vi "MARATHON_CHARGING1.vi"() -> ()   [LabVIEW 2018]
uses:
  <userlib>/LV-Link3/PolySubVIs/DtOLTimingSetInput.vi
  <userlib>/LV-Link3/PolySubVIs/DtOLReadMultiple2D.vi
panel:
  out "Waveform Graph":dbl[](graph)
  out "Transition Time":dbl format="%<%H:%M:%S>t"
  out "Array":bool[](array[boolean])
  in  "Limit Batt Voltage":dbl[](array[numeric]) format="%_4g"
  in  "Limit Cell Voltage":dbl[](array[numeric]) format="%_3g"
  out "x+y 2":dbl[](array[numeric])
  out "x+y":dbl[](array[knob]) scale=0.0..32.0
  out "Time 20":dbl format="%<%H:%M:%S>t"
  out "Time 19":dbl format="%<%H:%M:%S>t"
  out "Time 18":dbl format="%<%H:%M:%S>t"
  out "Time 17":dbl format="%<%H:%M:%S>t"
  out "Time 16":dbl format="%<%H:%M:%S>t"
  out "Time 15":dbl format="%<%H:%M:%S>t"
  out "Time 14":dbl format="%<%H:%M:%S>t"
  out "Time 13":dbl format="%<%H:%M:%S>t"
  out "Time 12":dbl format="%<%H:%M:%S>t"
  out "Time 11":dbl format="%<%H:%M:%S>t"
  out "Time 10":dbl format="%<%H:%M:%S>t"
  out "Time 9":dbl format="%<%H:%M:%S>t"
  out "Time 8":dbl format="%<%H:%M:%S>t"
  out "Time 7":dbl format="%<%H:%M:%S>t"
  out "Time 6":dbl format="%<%H:%M:%S>t"
  out "Time 5":dbl format="%<%H:%M:%S>t"
  out "Time 4":dbl format="%<%H:%M:%S>t"
  out "Time 3":dbl format="%<%H:%M:%S>t"
  out "Time 2":dbl format="%<%H:%M:%S>t"
  out "Time 1":dbl format="%<%H:%M:%S>t"
  out "CELL #19":bool[](array[boolean])
  out "CELL #20":bool[](array[boolean])
  out "CELL #18":bool[](array[boolean])
  out "CELL #17":bool[](array[boolean])
  out "CELL #16":bool[](array[boolean])
  out "CELL #15":bool[](array[boolean])
  out "CELL #14":bool[](array[boolean])
  out "CELL #13":bool[](array[boolean])
  out "CELL #12":bool[](array[boolean])
  out "CELL #11":bool[](array[boolean])
  out "CELL #10":bool[](array[boolean])
  out "CELL #9":bool[](array[boolean])
  out "CELL #8":bool[](array[boolean])
  out "CELL #7":bool[](array[boolean])
  out "CELL #6":bool[](array[boolean])
  out "CELL #5":bool[](array[boolean])
  out "CELL #4":bool[](array[boolean])
  out "CELL #3":bool[](array[boolean])
  out "CELL #2":bool[](array[boolean])
  out "CELL #1":bool[](array[boolean])
  out "VOLT # 20":dbl[](array[numeric])
  out "VOLT # 19":dbl[](array[numeric])
  out "VOLT # 18":dbl[](array[numeric])
  out "VOLT # 17":dbl[](array[numeric])
  out "VOLT # 16":dbl[](array[numeric])
  out "VOLT # 15":dbl[](array[numeric])
  out "VOLT # 14":dbl[](array[numeric])
  out "VOLT # 13":dbl[](array[numeric])
  out "VOLT # 12":dbl[](array[numeric])
  out "VOLT # 11":dbl[](array[numeric])
  out "VOLT # 10":dbl[](array[numeric])
  out "VOLT # 9":dbl[](array[numeric])
  out "VOLT # 8":dbl[](array[numeric])
  out "VOLT # 7":dbl[](array[numeric])
  out "VOLT # 6":dbl[](array[numeric])
  out "VOLT # 5":dbl[](array[numeric])
  out "VOLT # 4":dbl[](array[numeric])
  out "VOLT # 3":dbl[](array[numeric])
  out "VOLT # 2":dbl[](array[numeric])
  out "VOLT # 1":dbl[](array[numeric])
  in  "POWER":bool caption="START"
  in  "stop":bool
  # "FLUKE"
  # "179 Multimeter"
  # "28.56789 VOLTS"
  # "Hold"
  # "Range"
  # "ON"
  # "SuperMasterCharger"
  # "R"
  # "mV"
  # "Current"
  # "Time"
  # "000.7"
  # "04:56"
  # "D"
  # "V--"
  # "20 CELLS"
  # "Voltage"
  # "A--"
  # "OFF"
  # "STATUS"
  # "CHARGING"
  # "WATER"
  # "Jfm"
  # "ACID"
  # "1"
  # "Run"
  # "2"
  # "3"
  # "M"
  # "T"
  # "4"
  # "6"
  # "B"
  # "ST"
  # "5"
  # "CU"
  # "SAFT"
  # "8"
  # "OPT"
  # "V"
  # "RST"
  # "7"
  # "9"
  # "Vie"
  # "FN"
  # "ENT"
  # "0"
  # "C"
  # "P"
  # "POWER"
  # "Harness"
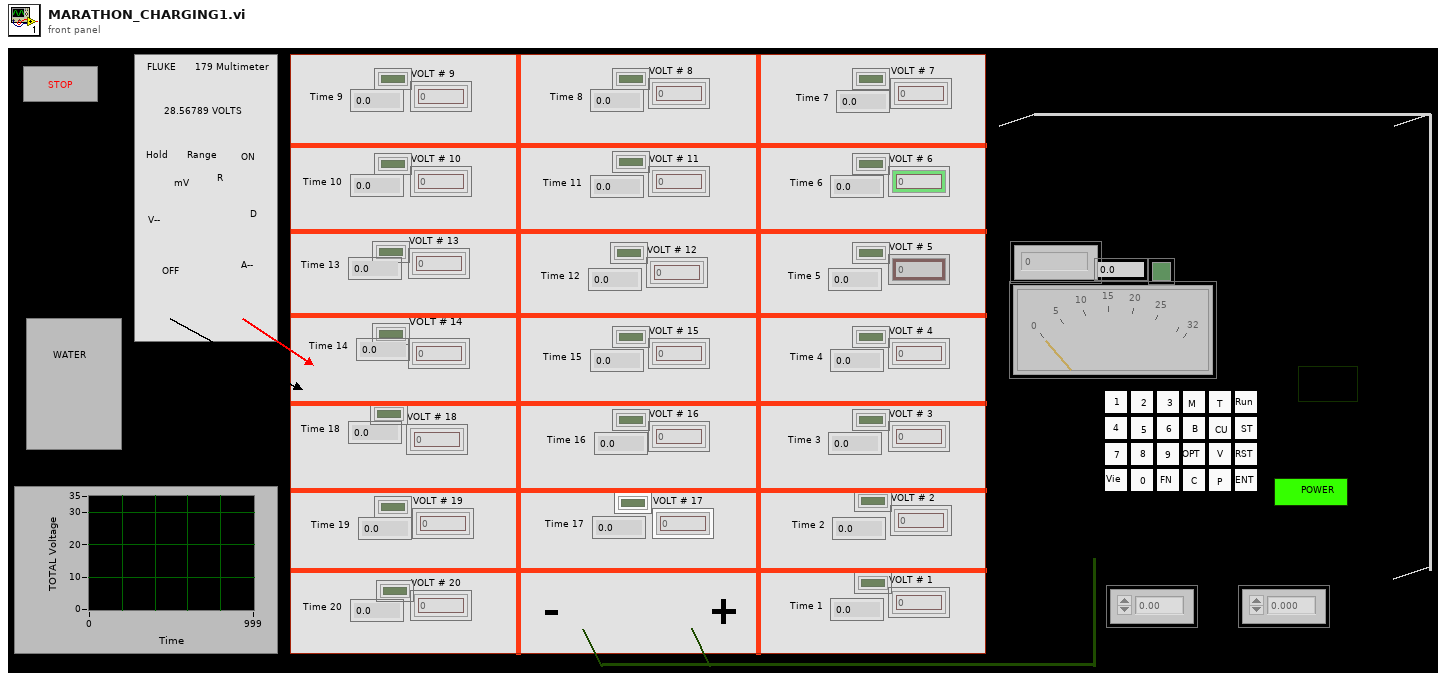
[diagram p1: front panel]
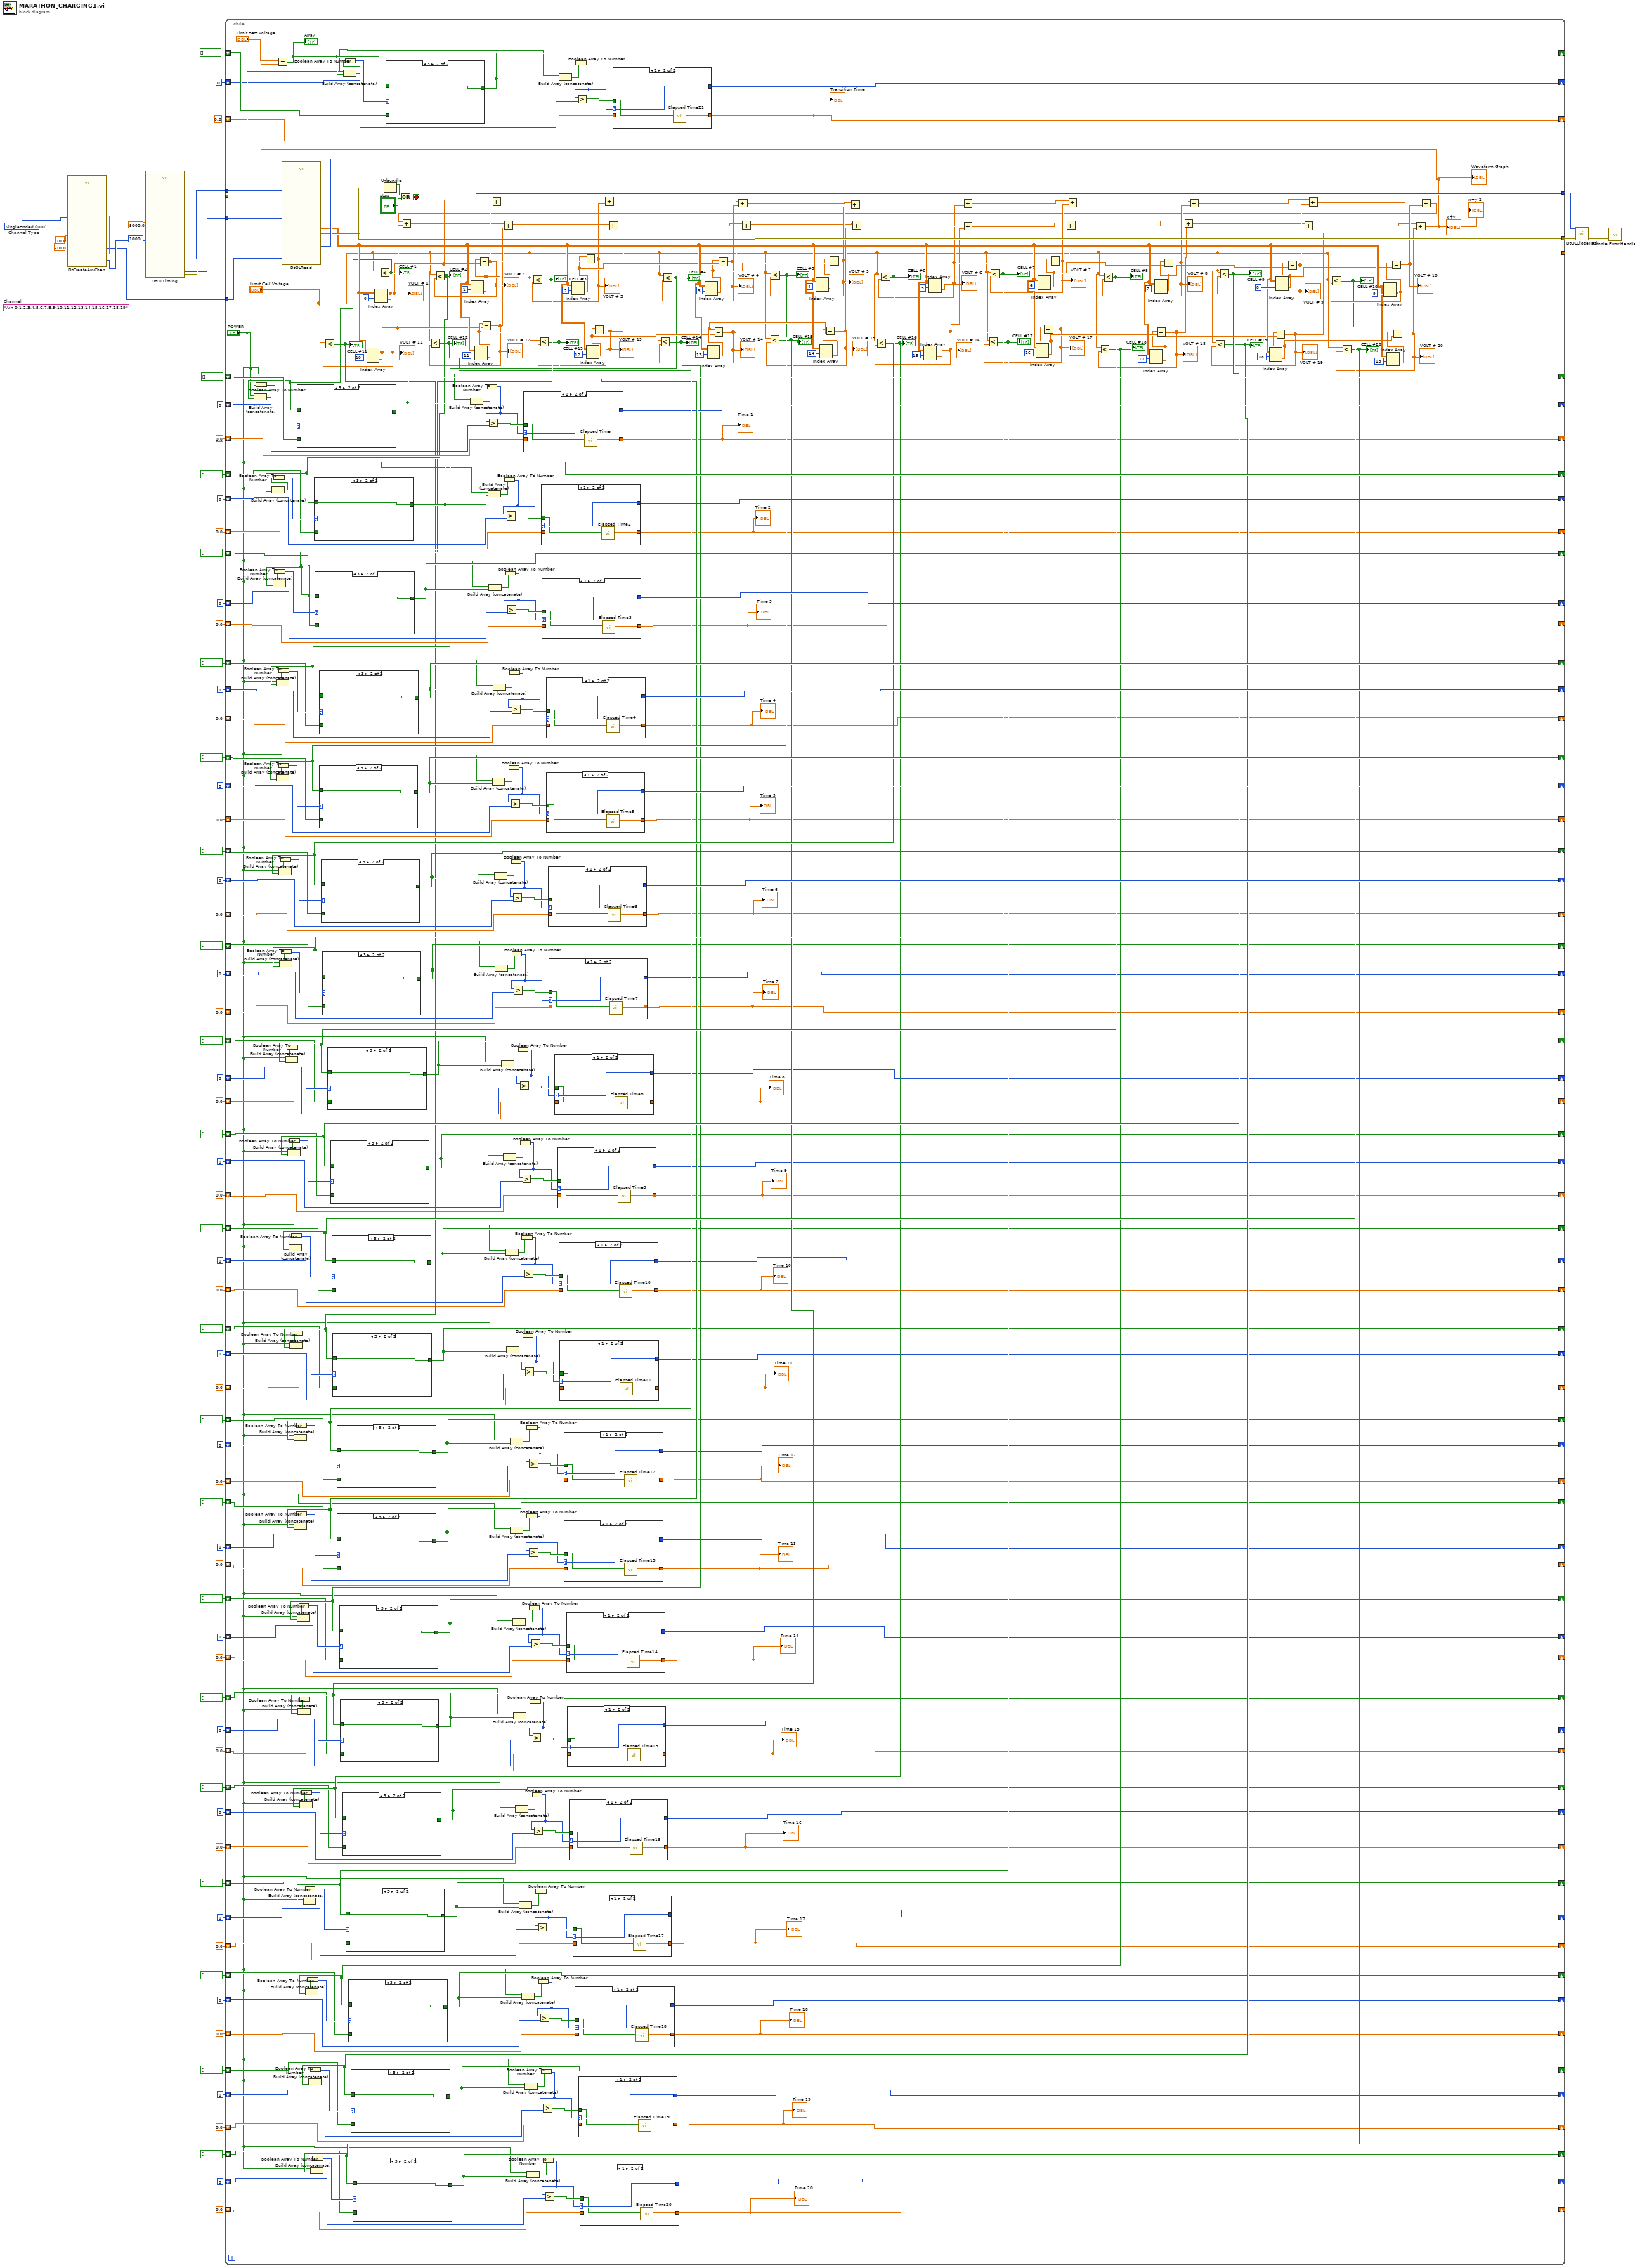
[diagram p0: block diagram]
diagram:
  w78 = 100 items=["Differential"=101, "SingleEnded"=100]  # Channel Type
  w75 = "Ain 0,1,2,3,4,5,6,7,8,9,10,11,12,13,14,15,16,17,18,19"  # Channel
  n1 = call <userlib>:"DtCreateAinChan.vi"("Channel Type"=w78, "Range Min"=-10.0, "Range Max"=10.0, "Channel"=w75) -> ("Task out"=w65:i32, "Actual Number of Channels"=w64:u32, "error out"=w74:errorcluster)  [unwired: 9 in]
  n2 = call-poly <userlib>:"DtOLTiming.vi"("Samples Per Channel"=u32 1000, "error in (no error)"=w74, "Sample Freq (Hz)"=5000.0, "Task in"=w65) -> ("error out"=w71:errorcluster, "Buffer Size"=w70:u32, "Task out"=w69:i32)  [unwired: 4 in, 1 out]
  n3 = while {
    tunnel: w71 -> [w418]
    tunnel: w70 -> [w416]
    tunnel: w69 -> [w417]
    tunnel: [w413] -> w68
    tunnel: [w414] -> w67
    tunnel: w64 -> [w412]
    shift-right: [w271] -> _
    shift-left: bool[] [] -> [w370]
    shift-right: [w230] -> _
    shift-left: u32 0 -> [w369]
    shift-right: [w117] -> _
    shift-left: 0.0 ("Elapsed Time (s)") -> [w368]
    shift-right: [w270] -> _
    shift-left: bool[] [] -> [w269]
    shift-right: [w267] -> _
    shift-left: u32 0 -> [w266]
    shift-right: [w99] -> _
    shift-left: 0.0 ("Elapsed Time (s)") -> [w265]
    shift-right: [w264] -> _
    shift-left: bool[] [] -> [w263]
    shift-right: [w262] -> _
    shift-left: u32 0 -> [w261]
    shift-right: [w98] -> _
    shift-left: 0.0 ("Elapsed Time (s)") -> [w260]
    shift-right: [w259] -> _
    shift-left: bool[] [] -> [w258]
    shift-right: [w257] -> _
    shift-left: u32 0 -> [w256]
    shift-right: [w96] -> _
    shift-left: 0.0 ("Elapsed Time (s)") -> [w255]
    shift-right: [w254] -> _
    shift-left: bool[] [] -> [w252]
    shift-right: [w253] -> _
    shift-left: u32 0 -> [w251]
    shift-right: [w95] -> _
    shift-left: 0.0 ("Elapsed Time (s)") -> [w250]
    shift-right: [w249] -> _
    shift-left: bool[] [] -> [w248]
    shift-right: [w247] -> _
    shift-left: u32 0 -> [w246]
    shift-right: [w94] -> _
    shift-left: 0.0 ("Elapsed Time (s)") -> [w245]
    shift-right: [w222] -> _
    shift-left: bool[] [] -> [w221]
    shift-right: [w220] -> _
    shift-left: u32 0 -> [w219]
    shift-right: [w93] -> _
    shift-left: 0.0 ("Elapsed Time (s)") -> [w218]
    shift-right: [w217] -> _
    shift-left: bool[] [] -> [w191]
    shift-right: [w216] -> _
    shift-left: u32 0 -> [w190]
    shift-right: [w92] -> _
    shift-left: 0.0 ("Elapsed Time (s)") -> [w189]
    shift-right: [w215] -> _
    shift-left: bool[] [] -> [w188]
    shift-right: [w214] -> _
    shift-left: u32 0 -> [w187]
    shift-right: [w91] -> _
    shift-left: 0.0 ("Elapsed Time (s)") -> [w186]
    shift-right: [w213] -> _
    shift-left: bool[] [] -> [w185]
    shift-right: [w212] -> _
    shift-left: u32 0 -> [w184]
    shift-right: [w90] -> _
    shift-left: 0.0 ("Elapsed Time (s)") -> [w183]
    shift-right: [w211] -> _
    shift-left: bool[] [] -> [w182]
    shift-right: [w210] -> _
    shift-left: u32 0 -> [w181]
    shift-right: [w89] -> _
    shift-left: 0.0 ("Elapsed Time (s)") -> [w180]
    shift-right: [w209] -> _
    shift-left: bool[] [] -> [w179]
    shift-right: [w208] -> _
    shift-left: u32 0 -> [w178]
    shift-right: [w88] -> _
    shift-left: 0.0 ("Elapsed Time (s)") -> [w177]
    shift-right: [w207] -> _
    shift-left: bool[] [] -> [w176]
    shift-right: [w206] -> _
    shift-left: u32 0 -> [w175]
    shift-right: [w87] -> _
    shift-left: 0.0 ("Elapsed Time (s)") -> [w174]
    shift-right: [w205] -> _
    shift-left: bool[] [] -> [w173]
    shift-right: [w204] -> _
    shift-left: u32 0 -> [w172]
    shift-right: [w86] -> _
    shift-left: 0.0 ("Elapsed Time (s)") -> [w171]
    shift-right: [w203] -> _
    shift-left: bool[] [] -> [w170]
    shift-right: [w202] -> _
    shift-left: u32 0 -> [w169]
    shift-right: [w85] -> _
    shift-left: 0.0 ("Elapsed Time (s)") -> [w168]
    shift-right: [w201] -> _
    shift-left: bool[] [] -> [w167]
    shift-right: [w200] -> _
    shift-left: u32 0 -> [w166]
    shift-right: [w84] -> _
    shift-left: 0.0 ("Elapsed Time (s)") -> [w165]
    shift-right: [w199] -> _
    shift-left: bool[] [] -> [w164]
    shift-right: [w198] -> _
    shift-left: u32 0 -> [w163]
    shift-right: [w83] -> _
    shift-left: 0.0 ("Elapsed Time (s)") -> [w162]
    shift-right: [w197] -> _
    shift-left: bool[] [] -> [w161]
    shift-right: [w196] -> _
    shift-left: u32 0 -> [w160]
    shift-right: [w82] -> _
    shift-left: 0.0 ("Elapsed Time (s)") -> [w159]
    shift-right: [w195] -> _
    shift-left: bool[] [] -> [w158]
    shift-right: [w194] -> _
    shift-left: u32 0 -> [w157]
    shift-right: [w81] -> _
    shift-left: 0.0 ("Elapsed Time (s)") -> [w156]
    shift-right: [w193] -> _
    shift-left: bool[] [] -> [w155]
    shift-right: [w192] -> _
    shift-left: u32 0 -> [w154]
    shift-right: [w80] -> _
    shift-left: 0.0 ("Elapsed Time (s)") -> [w153]
    tunnel: ["Limit Cell Voltage"] -> _
    shift-right: [w105] -> _
    shift-left: bool[] [] -> [w104]
    shift-right: [w102] -> _
    shift-left: u32 0 -> [w101]
    shift-right: [w97] -> _
    shift-left: 0.0 ("Elapsed Time (s)") -> [w100]
    stop <- w390 stop-if-true
    n4 = call-poly <userlib>:"DtOLRead.vi"("Number Chan to Read"=w412, "Buffer size"=w416, "error in (no error)"=w418, "Task in"=w417) -> ("error out"=w413:errorcluster, "2D Data out"=w389:dbl[][], "Task out"=w414:i32)  [unwired: 3 in, 2 out]
    n5 = Index Array(array=w389, index (row)=10) -> (element=w115:dbl[])  [unwired: 1 in]
    "VOLT # 11" <- w115
    n6 = Less?(x="Limit Cell Voltage", y=w115) -> (x < y?=w233:bool[])
    "CELL #11" <- w233
    n7 = Build Array (concatenate)("POWER", w233) -> (w318:bool[])
    n8 = Boolean Array To Number(Boolean array=w318) -> (number=w317:u32)
    n9 = case shown="3" w317 {
      tunnel: w233 -> [_ w495]
      tunnel: [w494 w495] -> w211
      tunnel: w182 -> [w494 _]
      frame 0, Default {
      }
      frame 3 {
      }
    }
    n10 = Index Array(array=w389, index (row)=0) -> (element=w152:dbl[])  [unwired: 1 in]
    "VOLT # 1" <- w152
    n11 = Less?(x="Limit Cell Voltage", y=w152) -> (x < y?=w244:bool[])
    "CELL #1" <- w244
    n12 = Build Array (concatenate)("POWER", w244) -> (w367:bool[])
    n13 = Boolean Array To Number(Boolean array=w367) -> (number=w366:u32)
    n14 = case shown="3" w366 {
      tunnel: w244 -> [_ w565]
      tunnel: [w564 w565] -> w271
      tunnel: w370 -> [w564 _]
      frame 0, Default {
      }
      frame 3 {
      }
    }
    n15 = Unbundle "Unbundle"(w413) -> ("status"=w415:bool)  [unwired: 2 out]
    n16 = Or(x=w415, y="stop") -> (x .or. y?=w390:bool)
    n17 = Build Array (concatenate)("POWER", w271) -> (w372:bool[])
    n18 = Index Array(array=w389, index (row)=1) -> (element=w388:dbl[])  [unwired: 1 in]
    n19 = Index Array(array=w389, index (row)=11) -> (element=w380:dbl[])  [unwired: 1 in]
    n20 = Subtract(x=w388, y=w152) -> (x-y=w151:dbl[])
    "VOLT # 2" <- w151
    n21 = Less?(x="Limit Cell Voltage", y=w151) -> (x < y?=w243:bool[])
    "CELL #2" <- w243
    n22 = Build Array (concatenate)("POWER", w243) -> (w268:bool[])
    n23 = Boolean Array To Number(Boolean array=w268) -> (number=w362:u32)
    n24 = case shown="3" w362 {
      tunnel: w243 -> [_ w558]
      tunnel: [w557 w558] -> w270
      tunnel: w269 -> [w557 _]
      frame 0, Default {
      }
      frame 3 {
      }
    }
    n25 = Subtract(x=w380, y=w115) -> (x-y=w133:dbl[])
    "VOLT # 12" <- w133
    n26 = Less?(x="Limit Cell Voltage", y=w133) -> (x < y?=w232:bool[])
    "CELL #12" <- w232
    n27 = Build Array (concatenate)("POWER", w232) -> (w313:bool[])
    n28 = Boolean Array To Number(Boolean array=w313) -> (number=w312:u32)
    n29 = case shown="3" w312 {
      tunnel: w232 -> [_ w488]
      tunnel: [w487 w488] -> w209
      tunnel: w179 -> [w487 _]
      frame 0, Default {
      }
      frame 3 {
      }
    }
    n30 = Boolean Array To Number(Boolean array=w372) -> (number=w371:u32)
    n31 = Greater?(x=w371, y=w369) -> (0:w373:bool)
    n32 = Build Array (concatenate)("POWER", w270) -> (w364:bool[])
    n33 = Add(x=w152, y=w151) -> (x+y=w150:dbl[])
    n34 = Boolean Array To Number(Boolean array=w364) -> (number=w363:u32)
    n35 = Greater?(x=w363, y=w266) -> (0:w365:bool)
    n36 = Build Array (concatenate)("POWER", w211) -> (w320:bool[])
    n37 = Build Array (concatenate)("POWER", w209) -> (w315:bool[])
    n38 = Boolean Array To Number(Boolean array=w320) -> (number=w319:u32)
    n39 = Greater?(x=w319, y=w181) -> (0:w321:bool)
    n40 = case shown="1" w371 {
      selector: w371 -> [w560 w562]
      tunnel: [w559 w563] -> w117
      tunnel: w368 -> [w559 _]
      tunnel: [w560 w562] -> w230
      tunnel: w373 -> [_ w561]
      frame 0, Default {
      }
      frame 1 {
        n41 = call "Elapsed Time"("Reset"=w561) -> ("Elapsed Time (s)"=w563:dbl)  [unwired: 11 in, 7 out]
      }
    }
    "Time 1" <- w117
    n42 = Boolean Array To Number(Boolean array=w315) -> (number=w314:u32)
    n43 = Greater?(x=w314, y=w178) -> (0:w316:bool)
    n44 = case shown="1" w363 {
      selector: w363 -> [w553 w555]
      tunnel: [w552 w556] -> w99
      tunnel: w265 -> [w552 _]
      tunnel: [w553 w555] -> w267
      tunnel: w365 -> [_ w554]
      frame 0, Default {
      }
      frame 1 {
        n45 = call "Elapsed Time2"("Reset"=w554) -> ("Elapsed Time (s)"=w556:dbl)  [unwired: 11 in, 7 out]
      }
    }
    "Time 2" <- w99
    n46 = case shown="1" w319 {
      selector: w319 -> [w490 w492]
      tunnel: [w489 w493] -> w89
      tunnel: w180 -> [w489 _]
      tunnel: [w490 w492] -> w210
      tunnel: w321 -> [_ w491]
      frame 0, Default {
      }
      frame 1 {
        n47 = call "Elapsed Time11"("Reset"=w491) -> ("Elapsed Time (s)"=w493:dbl)  [unwired: 11 in, 7 out]
      }
    }
    "Time 11" <- w89
    n48 = case shown="1" w314 {
      selector: w314 -> [w483 w485]
      tunnel: [w482 w486] -> w88
      tunnel: w177 -> [w482 _]
      tunnel: [w483 w485] -> w208
      tunnel: w316 -> [_ w484]
      frame 0, Default {
      }
      frame 1 {
        n49 = call "Elapsed Time12"("Reset"=w484) -> ("Elapsed Time (s)"=w486:dbl)  [unwired: 11 in, 7 out]
      }
    }
    "Time 12" <- w88
    n50 = Index Array(array=w389, index (row)=2) -> (element=w387:dbl[])  [unwired: 1 in]
    n51 = Subtract(x=w387, y=w388) -> (x-y=w149:dbl[])
    "VOLT # 3" <- w149
    n52 = Less?(x="Limit Cell Voltage", y=w149) -> (x < y?=w242:bool[])
    "CELL #3" <- w242
    n53 = Build Array (concatenate)("POWER", w242) -> (w358:bool[])
    n54 = Boolean Array To Number(Boolean array=w358) -> (number=w357:u32)
    n55 = case shown="3" w357 {
      tunnel: w242 -> [_ w551]
      tunnel: [w550 w551] -> w264
      tunnel: w263 -> [w550 _]
      frame 0, Default {
      }
      frame 3 {
      }
    }
    n56 = Build Array (concatenate)("POWER", w264) -> (w360:bool[])
    n57 = Boolean Array To Number(Boolean array=w360) -> (number=w359:u32)
    n58 = Greater?(x=w359, y=w261) -> (0:w361:bool)
    n59 = case shown="1" w359 {
      selector: w359 -> [w546 w548]
      tunnel: [w545 w549] -> w98
      tunnel: w260 -> [w545 _]
      tunnel: [w546 w548] -> w262
      tunnel: w361 -> [_ w547]
      frame 0, Default {
      }
      frame 1 {
        n60 = call "Elapsed Time3"("Reset"=w547) -> ("Elapsed Time (s)"=w549:dbl)  [unwired: 11 in, 7 out]
      }
    }
    "Time 3" <- w98
    n61 = Index Array(array=w389, index (row)=12) -> (element=w241:dbl[])  [unwired: 1 in]
    n62 = Subtract(x=w241, y=w380) -> (x-y=w131:dbl[])
    "VOLT # 13" <- w131
    n63 = Less?(x="Limit Cell Voltage", y=w131) -> (x < y?=w231:bool[])
    "CELL #13" <- w231
    n64 = Build Array (concatenate)("POWER", w231) -> (w308:bool[])
    n65 = Boolean Array To Number(Boolean array=w308) -> (number=w307:u32)
    n66 = case shown="3" w307 {
      tunnel: w231 -> [_ w481]
      tunnel: [w480 w481] -> w207
      tunnel: w176 -> [w480 _]
      frame 0, Default {
      }
      frame 3 {
      }
    }
    n67 = Build Array (concatenate)("POWER", w207) -> (w310:bool[])
    n68 = Boolean Array To Number(Boolean array=w310) -> (number=w309:u32)
    n69 = Greater?(x=w309, y=w175) -> (0:w311:bool)
    n70 = case shown="1" w309 {
      selector: w309 -> [w476 w478]
      tunnel: [w475 w479] -> w87
      tunnel: w174 -> [w475 _]
      tunnel: [w476 w478] -> w206
      tunnel: w311 -> [_ w477]
      frame 0, Default {
      }
      frame 1 {
        n71 = call "Elapsed Time13"("Reset"=w477) -> ("Elapsed Time (s)"=w479:dbl)  [unwired: 11 in, 7 out]
      }
    }
    "Time 13" <- w87
    n72 = Add(x=w150, y=w149) -> (x+y=w148:dbl[])
    n73 = Index Array(array=w389, index (row)=3) -> (element=w386:dbl[])  [unwired: 1 in]
    n74 = Index Array(array=w389, index (row)=13) -> (element=w379:dbl[])  [unwired: 1 in]
    n75 = Subtract(x=w379, y=w241) -> (x-y=w129:dbl[])
    "VOLT # 14" <- w129
    n76 = Less?(x="Limit Cell Voltage", y=w129) -> (x < y?=w229:bool[])
    "CELL #14" <- w229
    n77 = Build Array (concatenate)("POWER", w229) -> (w303:bool[])
    n78 = Boolean Array To Number(Boolean array=w303) -> (number=w302:u32)
    n79 = case shown="3" w302 {
      tunnel: w229 -> [_ w474]
      tunnel: [w473 w474] -> w205
      tunnel: w173 -> [w473 _]
      frame 0, Default {
      }
      frame 3 {
      }
    }
    n80 = Build Array (concatenate)("POWER", w205) -> (w305:bool[])
    n81 = Boolean Array To Number(Boolean array=w305) -> (number=w304:u32)
    n82 = Greater?(x=w304, y=w172) -> (0:w306:bool)
    n83 = case shown="1" w304 {
      selector: w304 -> [w469 w471]
      tunnel: [w468 w472] -> w86
      tunnel: w171 -> [w468 _]
      tunnel: [w469 w471] -> w204
      tunnel: w306 -> [_ w470]
      frame 0, Default {
      }
      frame 1 {
        n84 = call "Elapsed Time14"("Reset"=w470) -> ("Elapsed Time (s)"=w472:dbl)  [unwired: 11 in, 7 out]
      }
    }
    "Time 14" <- w86
    n85 = Subtract(x=w386, y=w387) -> (x-y=w147:dbl[])
    "VOLT # 4" <- w147
    n86 = Less?(x="Limit Cell Voltage", y=w147) -> (x < y?=w240:bool[])
    "CELL #4" <- w240
    n87 = Build Array (concatenate)("POWER", w240) -> (w353:bool[])
    n88 = Boolean Array To Number(Boolean array=w353) -> (number=w352:u32)
    n89 = case shown="3" w352 {
      tunnel: w240 -> [_ w544]
      tunnel: [w543 w544] -> w259
      tunnel: w258 -> [w543 _]
      frame 0, Default {
      }
      frame 3 {
      }
    }
    n90 = Build Array (concatenate)("POWER", w259) -> (w355:bool[])
    n91 = Boolean Array To Number(Boolean array=w355) -> (number=w354:u32)
    n92 = Greater?(x=w354, y=w256) -> (0:w356:bool)
    n93 = case shown="1" w354 {
      selector: w354 -> [w539 w541]
      tunnel: [w538 w542] -> w96
      tunnel: w255 -> [w538 _]
      tunnel: [w539 w541] -> w257
      tunnel: w356 -> [_ w540]
      frame 0, Default {
      }
      frame 1 {
        n94 = call "Elapsed Time4"("Reset"=w540) -> ("Elapsed Time (s)"=w542:dbl)  [unwired: 11 in, 7 out]
      }
    }
    "Time 4" <- w96
    n95 = Add(x=w148, y=w147) -> (x+y=w146:dbl[])
    n96 = Index Array(array=w389, index (row)=4) -> (element=w385:dbl[])  [unwired: 1 in]
    n97 = Index Array(array=w389, index (row)=14) -> (element=w378:dbl[])  [unwired: 1 in]
    n98 = Subtract(x=w378, y=w379) -> (x-y=w127:dbl[])
    "VOLT # 15" <- w127
    n99 = Less?(x="Limit Cell Voltage", y=w127) -> (x < y?=w228:bool[])
    "CELL #15" <- w228
    n100 = Build Array (concatenate)("POWER", w228) -> (w298:bool[])
    n101 = Boolean Array To Number(Boolean array=w298) -> (number=w297:u32)
    n102 = case shown="3" w297 {
      tunnel: w228 -> [_ w467]
      tunnel: [w466 w467] -> w203
      tunnel: w170 -> [w466 _]
      frame 0, Default {
      }
      frame 3 {
      }
    }
    n103 = Build Array (concatenate)("POWER", w203) -> (w300:bool[])
    n104 = Boolean Array To Number(Boolean array=w300) -> (number=w299:u32)
    n105 = Greater?(x=w299, y=w169) -> (0:w301:bool)
    n106 = case shown="1" w299 {
      selector: w299 -> [w462 w464]
      tunnel: [w461 w465] -> w85
      tunnel: w168 -> [w461 _]
      tunnel: [w462 w464] -> w202
      tunnel: w301 -> [_ w463]
      frame 0, Default {
      }
      frame 1 {
        n107 = call "Elapsed Time15"("Reset"=w463) -> ("Elapsed Time (s)"=w465:dbl)  [unwired: 11 in, 7 out]
      }
    }
    "Time 15" <- w85
    n108 = Subtract(x=w385, y=w386) -> (x-y=w145:dbl[])
    "VOLT # 5" <- w145
    n109 = Less?(x="Limit Cell Voltage", y=w145) -> (x < y?=w239:bool[])
    "CELL #5" <- w239
    n110 = Build Array (concatenate)("POWER", w239) -> (w348:bool[])
    n111 = Boolean Array To Number(Boolean array=w348) -> (number=w347:u32)
    n112 = case shown="3" w347 {
      tunnel: w239 -> [_ w537]
      tunnel: [w536 w537] -> w254
      tunnel: w252 -> [w536 _]
      frame 0, Default {
      }
      frame 3 {
      }
    }
    n113 = Build Array (concatenate)("POWER", w254) -> (w350:bool[])
    n114 = Boolean Array To Number(Boolean array=w350) -> (number=w349:u32)
    n115 = Greater?(x=w349, y=w251) -> (0:w351:bool)
    n116 = case shown="1" w349 {
      selector: w349 -> [w532 w534]
      tunnel: [w531 w535] -> w95
      tunnel: w250 -> [w531 _]
      tunnel: [w532 w534] -> w253
      tunnel: w351 -> [_ w533]
      frame 0, Default {
      }
      frame 1 {
        n117 = call "Elapsed Time5"("Reset"=w533) -> ("Elapsed Time (s)"=w535:dbl)  [unwired: 11 in, 7 out]
      }
    }
    "Time 5" <- w95
    n118 = Add(x=w146, y=w145) -> (x+y=w144:dbl[])
    n119 = Index Array(array=w389, index (row)=15) -> (element=w114:dbl[])  [unwired: 1 in]
    "VOLT # 16" <- w114
    n120 = Less?(x="Limit Cell Voltage", y=w114) -> (x < y?=w227:bool[])
    "CELL #16" <- w227
    n121 = Build Array (concatenate)("POWER", w227) -> (w293:bool[])
    n122 = Boolean Array To Number(Boolean array=w293) -> (number=w292:u32)
    n123 = case shown="3" w292 {
      tunnel: w227 -> [_ w460]
      tunnel: [w459 w460] -> w201
      tunnel: w167 -> [w459 _]
      frame 0, Default {
      }
      frame 3 {
      }
    }
    n124 = Build Array (concatenate)("POWER", w201) -> (w295:bool[])
    n125 = Boolean Array To Number(Boolean array=w295) -> (number=w294:u32)
    n126 = Greater?(x=w294, y=w166) -> (0:w296:bool)
    n127 = case shown="1" w294 {
      selector: w294 -> [w455 w457]
      tunnel: [w454 w458] -> w84
      tunnel: w165 -> [w454 _]
      tunnel: [w455 w457] -> w200
      tunnel: w296 -> [_ w456]
      frame 0, Default {
      }
      frame 1 {
        n128 = call "Elapsed Time16"("Reset"=w456) -> ("Elapsed Time (s)"=w458:dbl)  [unwired: 11 in, 7 out]
      }
    }
    "Time 16" <- w84
    n129 = Index Array(array=w389, index (row)=5) -> (element=w116:dbl[])  [unwired: 1 in]
    "VOLT # 6" <- w116
    n130 = Less?(x="Limit Cell Voltage", y=w116) -> (x < y?=w238:bool[])
    "CELL #6" <- w238
    n131 = Build Array (concatenate)("POWER", w238) -> (w343:bool[])
    n132 = Boolean Array To Number(Boolean array=w343) -> (number=w342:u32)
    n133 = case shown="3" w342 {
      tunnel: w238 -> [_ w530]
      tunnel: [w529 w530] -> w249
      tunnel: w248 -> [w529 _]
      frame 0, Default {
      }
      frame 3 {
      }
    }
    n134 = Build Array (concatenate)("POWER", w249) -> (w345:bool[])
    n135 = Boolean Array To Number(Boolean array=w345) -> (number=w344:u32)
    n136 = Greater?(x=w344, y=w246) -> (0:w346:bool)
    n137 = case shown="1" w344 {
      selector: w344 -> [w525 w527]
      tunnel: [w524 w528] -> w94
      tunnel: w245 -> [w524 _]
      tunnel: [w525 w527] -> w247
      tunnel: w346 -> [_ w526]
      frame 0, Default {
      }
      frame 1 {
        n138 = call "Elapsed Time6"("Reset"=w526) -> ("Elapsed Time (s)"=w528:dbl)  [unwired: 11 in, 7 out]
      }
    }
    "Time 6" <- w94
    n139 = Add(x=w144, y=w116) -> (x+y=w143:dbl[])
    n140 = Index Array(array=w389, index (row)=16) -> (element=w377:dbl[])  [unwired: 1 in]
    n141 = Index Array(array=w389, index (row)=6) -> (element=w384:dbl[])  [unwired: 1 in]
    n142 = Subtract(x=w377, y=w114) -> (x-y=w124:dbl[])
    "VOLT # 17" <- w124
    n143 = Less?(x="Limit Cell Voltage", y=w124) -> (x < y?=w226:bool[])
    "CELL #17" <- w226
    n144 = Build Array (concatenate)("POWER", w226) -> (w288:bool[])
    n145 = Boolean Array To Number(Boolean array=w288) -> (number=w287:u32)
    n146 = case shown="3" w287 {
      tunnel: w226 -> [_ w453]
      tunnel: [w452 w453] -> w199
      tunnel: w164 -> [w452 _]
      frame 0, Default {
      }
      frame 3 {
      }
    }
    n147 = Build Array (concatenate)("POWER", w199) -> (w290:bool[])
    n148 = Boolean Array To Number(Boolean array=w290) -> (number=w289:u32)
    n149 = Greater?(x=w289, y=w163) -> (0:w291:bool)
    n150 = case shown="1" w289 {
      selector: w289 -> [w448 w450]
      tunnel: [w447 w451] -> w83
      tunnel: w162 -> [w447 _]
      tunnel: [w448 w450] -> w198
      tunnel: w291 -> [_ w449]
      frame 0, Default {
      }
      frame 1 {
        n151 = call "Elapsed Time17"("Reset"=w449) -> ("Elapsed Time (s)"=w451:dbl)  [unwired: 11 in, 7 out]
      }
    }
    "Time 17" <- w83
    n152 = Subtract(x=w384, y=w116) -> (x-y=w142:dbl[])
    "VOLT # 7" <- w142
    n153 = Less?(x="Limit Cell Voltage", y=w142) -> (x < y?=w237:bool[])
    "CELL #7" <- w237
    n154 = Build Array (concatenate)("POWER", w237) -> (w338:bool[])
    n155 = Boolean Array To Number(Boolean array=w338) -> (number=w337:u32)
    n156 = case shown="3" w337 {
      tunnel: w237 -> [_ w523]
      tunnel: [w522 w523] -> w222
      tunnel: w221 -> [w522 _]
      frame 0, Default {
      }
      frame 3 {
      }
    }
    n157 = Build Array (concatenate)("POWER", w222) -> (w340:bool[])
    n158 = Boolean Array To Number(Boolean array=w340) -> (number=w339:u32)
    n159 = Greater?(x=w339, y=w219) -> (0:w341:bool)
    n160 = case shown="1" w339 {
      selector: w339 -> [w518 w520]
      tunnel: [w517 w521] -> w93
      tunnel: w218 -> [w517 _]
      tunnel: [w518 w520] -> w220
      tunnel: w341 -> [_ w519]
      frame 0, Default {
      }
      frame 1 {
        n161 = call "Elapsed Time7"("Reset"=w519) -> ("Elapsed Time (s)"=w521:dbl)  [unwired: 11 in, 7 out]
      }
    }
    "Time 7" <- w93
    n162 = Add(x=w143, y=w142) -> (x+y=w141:dbl[])
    n163 = Index Array(array=w389, index (row)=17) -> (element=w376:dbl[])  [unwired: 1 in]
    n164 = Index Array(array=w389, index (row)=7) -> (element=w383:dbl[])  [unwired: 1 in]
    n165 = Subtract(x=w376, y=w377) -> (x-y=w122:dbl[])
    "VOLT # 18" <- w122
    n166 = Less?(x="Limit Cell Voltage", y=w122) -> (x < y?=w225:bool[])
    "CELL #18" <- w225
    n167 = Build Array (concatenate)("POWER", w225) -> (w283:bool[])
    n168 = Boolean Array To Number(Boolean array=w283) -> (number=w282:u32)
    n169 = case shown="3" w282 {
      tunnel: w225 -> [_ w446]
      tunnel: [w445 w446] -> w197
      tunnel: w161 -> [w445 _]
      frame 0, Default {
      }
      frame 3 {
      }
    }
    n170 = Build Array (concatenate)("POWER", w197) -> (w285:bool[])
    n171 = Boolean Array To Number(Boolean array=w285) -> (number=w284:u32)
    n172 = Greater?(x=w284, y=w160) -> (0:w286:bool)
    n173 = case shown="1" w284 {
      selector: w284 -> [w441 w443]
      tunnel: [w440 w444] -> w82
      tunnel: w159 -> [w440 _]
      tunnel: [w441 w443] -> w196
      tunnel: w286 -> [_ w442]
      frame 0, Default {
      }
      frame 1 {
        n174 = call "Elapsed Time18"("Reset"=w442) -> ("Elapsed Time (s)"=w444:dbl)  [unwired: 11 in, 7 out]
      }
    }
    "Time 18" <- w82
    n175 = Subtract(x=w383, y=w384) -> (x-y=w140:dbl[])
    "VOLT # 8" <- w140
    n176 = Less?(x="Limit Cell Voltage", y=w140) -> (x < y?=w236:bool[])
    "CELL #8" <- w236
    n177 = Build Array (concatenate)("POWER", w236) -> (w333:bool[])
    n178 = Boolean Array To Number(Boolean array=w333) -> (number=w332:u32)
    n179 = case shown="3" w332 {
      tunnel: w236 -> [_ w516]
      tunnel: [w515 w516] -> w217
      tunnel: w191 -> [w515 _]
      frame 0, Default {
      }
      frame 3 {
      }
    }
    n180 = Build Array (concatenate)("POWER", w217) -> (w335:bool[])
    n181 = Boolean Array To Number(Boolean array=w335) -> (number=w334:u32)
    n182 = Greater?(x=w334, y=w190) -> (0:w336:bool)
    n183 = case shown="1" w334 {
      selector: w334 -> [w511 w513]
      tunnel: [w510 w514] -> w92
      tunnel: w189 -> [w510 _]
      tunnel: [w511 w513] -> w216
      tunnel: w336 -> [_ w512]
      frame 0, Default {
      }
      frame 1 {
        n184 = call "Elapsed Time8"("Reset"=w512) -> ("Elapsed Time (s)"=w514:dbl)  [unwired: 11 in, 7 out]
      }
    }
    "Time 8" <- w92
    n185 = Add(x=w141, y=w140) -> (x+y=w139:dbl[])
    n186 = Index Array(array=w389, index (row)=18) -> (element=w375:dbl[])  [unwired: 1 in]
    n187 = Subtract(x=w375, y=w376) -> (x-y=w120:dbl[])
    "VOLT # 19" <- w120
    n188 = Less?(x="Limit Cell Voltage", y=w120) -> (x < y?=w224:bool[])
    "CELL #19" <- w224
    n189 = Build Array (concatenate)("POWER", w224) -> (w278:bool[])
    n190 = Boolean Array To Number(Boolean array=w278) -> (number=w277:u32)
    n191 = case shown="3" w277 {
      tunnel: w224 -> [_ w439]
      tunnel: [w438 w439] -> w195
      tunnel: w158 -> [w438 _]
      frame 0, Default {
      }
      frame 3 {
      }
    }
    n192 = Build Array (concatenate)("POWER", w195) -> (w280:bool[])
    n193 = Boolean Array To Number(Boolean array=w280) -> (number=w279:u32)
    n194 = Greater?(x=w279, y=w157) -> (0:w281:bool)
    n195 = case shown="1" w279 {
      selector: w279 -> [w434 w436]
      tunnel: [w433 w437] -> w81
      tunnel: w156 -> [w433 _]
      tunnel: [w434 w436] -> w194
      tunnel: w281 -> [_ w435]
      frame 0, Default {
      }
      frame 1 {
        n196 = call "Elapsed Time19"("Reset"=w435) -> ("Elapsed Time (s)"=w437:dbl)  [unwired: 11 in, 7 out]
      }
    }
    "Time 19" <- w81
    n197 = Index Array(array=w389, index (row)=8) -> (element=w382:dbl[])  [unwired: 1 in]
    n198 = Subtract(x=w382, y=w383) -> (x-y=w138:dbl[])
    "VOLT # 9" <- w138
    n199 = Less?(x="Limit Cell Voltage", y=w138) -> (x < y?=w235:bool[])
    "CELL #9" <- w235
    n200 = Build Array (concatenate)("POWER", w235) -> (w328:bool[])
    n201 = Boolean Array To Number(Boolean array=w328) -> (number=w327:u32)
    n202 = case shown="3" w327 {
      tunnel: w235 -> [_ w509]
      tunnel: [w508 w509] -> w215
      tunnel: w188 -> [w508 _]
      frame 0, Default {
      }
      frame 3 {
      }
    }
    n203 = Build Array (concatenate)("POWER", w215) -> (w330:bool[])
    n204 = Boolean Array To Number(Boolean array=w330) -> (number=w329:u32)
    n205 = Greater?(x=w329, y=w187) -> (0:w331:bool)
    n206 = case shown="1" w329 {
      selector: w329 -> [w504 w506]
      tunnel: [w503 w507] -> w91
      tunnel: w186 -> [w503 _]
      tunnel: [w504 w506] -> w214
      tunnel: w331 -> [_ w505]
      frame 0, Default {
      }
      frame 1 {
        n207 = call "Elapsed Time9"("Reset"=w505) -> ("Elapsed Time (s)"=w507:dbl)  [unwired: 11 in, 7 out]
      }
    }
    "Time 9" <- w91
    n208 = Add(x=w139, y=w138) -> (x+y=w137:dbl[])
    n209 = Index Array(array=w389, index (row)=9) -> (element=w381:dbl[])  [unwired: 1 in]
    n210 = Less?(x="Limit Cell Voltage", y=w381) -> (x < y?=w234:bool[])
    "CELL #10" <- w234
    n211 = Build Array (concatenate)("POWER", w234) -> (w323:bool[])
    n212 = Boolean Array To Number(Boolean array=w323) -> (number=w322:u32)
    n213 = case shown="3" w322 {
      tunnel: w234 -> [_ w502]
      tunnel: [w501 w502] -> w213
      tunnel: w185 -> [w501 _]
      frame 0, Default {
      }
      frame 3 {
      }
    }
    n214 = Build Array (concatenate)("POWER", w213) -> (w325:bool[])
    n215 = Boolean Array To Number(Boolean array=w325) -> (number=w324:u32)
    n216 = Greater?(x=w324, y=w184) -> (0:w326:bool)
    n217 = case shown="1" w324 {
      selector: w324 -> [w497 w499]
      tunnel: [w496 w500] -> w90
      tunnel: w183 -> [w496 _]
      tunnel: [w497 w499] -> w212
      tunnel: w326 -> [_ w498]
      frame 0, Default {
      }
      frame 1 {
        n218 = call "Elapsed Time10"("Reset"=w498) -> ("Elapsed Time (s)"=w500:dbl)  [unwired: 11 in, 7 out]
      }
    }
    "Time 10" <- w90
    n219 = Index Array(array=w389, index (row)=19) -> (element=w374:dbl[])  [unwired: 1 in]
    n220 = Subtract(x=w381, y=w382) -> (x-y=w136:dbl[])
    "VOLT # 10" <- w136
    n221 = Subtract(x=w374, y=w375) -> (x-y=w118:dbl[])
    "VOLT # 20" <- w118
    n222 = Less?(x="Limit Cell Voltage", y=w118) -> (x < y?=w223:bool[])
    "CELL #20" <- w223
    n223 = Build Array (concatenate)("POWER", w223) -> (w273:bool[])
    n224 = Boolean Array To Number(Boolean array=w273) -> (number=w272:u32)
    n225 = case shown="3" w272 {
      tunnel: w223 -> [_ w432]
      tunnel: [w431 w432] -> w193
      tunnel: w155 -> [w431 _]
      frame 0, Default {
      }
      frame 3 {
      }
    }
    n226 = Build Array (concatenate)("POWER", w193) -> (w275:bool[])
    n227 = Boolean Array To Number(Boolean array=w275) -> (number=w274:u32)
    n228 = Greater?(x=w274, y=w154) -> (0:w276:bool)
    n229 = case shown="1" w274 {
      selector: w274 -> [w427 w429]
      tunnel: [w426 w430] -> w80
      tunnel: w153 -> [w426 _]
      tunnel: [w427 w429] -> w192
      tunnel: w276 -> [_ w428]
      frame 0, Default {
      }
      frame 1 {
        n230 = call "Elapsed Time20"("Reset"=w428) -> ("Elapsed Time (s)"=w430:dbl)  [unwired: 11 in, 7 out]
      }
    }
    "Time 20" <- w80
    n231 = Add(x=w137, y=w136) -> (x+y=w135:dbl[])
    n232 = Add(x=w135, y=w115) -> (x+y=w134:dbl[])
    n233 = Add(x=w134, y=w133) -> (x+y=w132:dbl[])
    n234 = Add(x=w132, y=w131) -> (x+y=w130:dbl[])
    n235 = Add(x=w130, y=w129) -> (x+y=w128:dbl[])
    n236 = Add(x=w128, y=w127) -> (x+y=w126:dbl[])
    n237 = Add(x=w126, y=w114) -> (x+y=w125:dbl[])
    n238 = Add(x=w125, y=w124) -> (x+y=w123:dbl[])
    n239 = Add(x=w123, y=w122) -> (x+y=w121:dbl[])
    n240 = Add(x=w121, y=w120) -> (x+y=w119:dbl[])
    n241 = Add(x=w119, y=w118) -> (x+y=w79:dbl[])
    "x+y" <- w79
    "x+y 2" <- w79
    "Waveform Graph" <- w79
    n242 = Equal?(x="Limit Batt Voltage", y=w79) -> (x = y?=w106:bool[])
    "Array" <- w106
    n243 = Build Array (concatenate)("POWER", w106) -> (w108:bool[])
    n244 = Boolean Array To Number(Boolean array=w108) -> (number=w107:u32)
    n245 = case shown="3" w107 {
      tunnel: w106 -> [_ w425]
      tunnel: [w424 w425] -> w105
      tunnel: w104 -> [w424 _]
      frame 0, Default {
      }
      frame 3 {
      }
    }
    n246 = Build Array (concatenate)("POWER", w105) -> (w110:bool[])
    n247 = Boolean Array To Number(Boolean array=w110) -> (number=w109:u32)
    n248 = Greater?(x=w109, y=w101) -> (0:w111:bool)
    n249 = case shown="1" w109 {
      selector: w109 -> [w420 w422]
      tunnel: [w419 w423] -> w97
      tunnel: w100 -> [w419 _]
      tunnel: [w420 w422] -> w102
      tunnel: w111 -> [_ w421]
      frame 0, Default {
      }
      frame 1 {
        n250 = call "Elapsed Time21"("Reset"=w421) -> ("Elapsed Time (s)"=w423:dbl)  [unwired: 11 in, 7 out]
      }
    }
    "Transition Time" <- w97
  }
  n251 = call <userlib>:"DtOLCloseTask.vi"("Error in"=w68, "Task in"=w67) -> ("Error Out"=w66:errorcluster)  [unwired: 9 in]
  n252 = call <vilib>:"Simple Error Handler.vi"("error in (no error)"=w66) -> ()  [unwired: 4 in, 5 out]
